vi "example_alignObjects1.vi"   [LabVIEW 2023]
uses:
  Ctrls/alignment.ctl
  BlockDiagram/BlockDiagram.lvclass
  C:/projects/TLC_Scripto/Source/AbstractDiagram/AbstractDiagram.lvclass
  Terminal/Terminal.lvclass
  C:/projects/TLC_Scripto/Source/GObject/GObject.lvclass
  AbstractDiagram/Read controlTerminals.vi
  TLC_Scripto.lvlib
  GObject/GObject.lvclass
types:
  T1 = typedef "TLC_Scripto.lvlib/alignment.ctl" = enum16{"Top", "Bottom", "Left", "Right", "Center"}
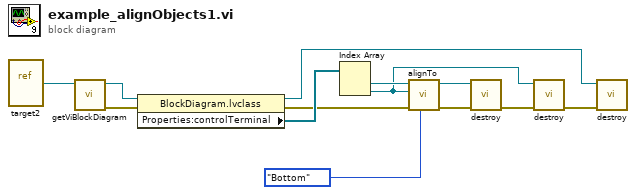
[diagram p0: block diagram]
diagram:
  n1 = vi-ref "target2.vi"() -> (w13:refnum<vi>)
  n2 = call "getViBlockDiagram.vi"("ViRef"=w13) -> ("error out"=w12:errorcluster, "topMostBlockDiagram"=w11:refnum<class "BlockDiagram.lvclass">)  [unwired: 9 in]
  n3 = property class="BlockDiagram.lvclass"(reference=w11, error in=w12) -> (reference out=w2:refnum<class "BlockDiagram.lvclass">, error out=w1:errorcluster, "Properties:controlTerminal"=w10:refnum<class "Terminal.lvclass">[])
  n4 = Index Array(array=w10) -> (element #1=w9:refnum<class "Terminal.lvclass">, element #2=w4:refnum<class "Terminal.lvclass">)  [unwired: 2 in]
  n5 = call "alignTo.vi"("alignment"=alignment."Bottom", "error in (no error)"=w1, "targetObj"=w4, "GObject in"=w9) -> ("error out"=w6:errorcluster, "GObject out"=w7:refnum<class "Terminal.lvclass">)  [unwired: 6 in]
  n6 = call-dynamic "destroy.vi"("Error In"=w6, "Generic In"=w7) -> ("Error Out"=w5:errorcluster)  [unwired: 9 in]
  n7 = call-dynamic "destroy.vi"("Error In"=w5, "Generic In"=w4) -> ("Error Out"=w3:errorcluster)  [unwired: 9 in]
  n8 = call-dynamic "destroy.vi"("Error In"=w3, "Generic In"=w2) -> ()  [unwired: 9 in, 1 out]
